vi "Check Duplicated Names.vi"(7 "Element Type":string, 8 "errors in":refnum<class "MultiErrors.lvclass">, 11 "Names":string[](array[string])) -> (0 "errors out":refnum<class "MultiErrors.lvclass">)   [LabVIEW 2020, in "VolatusConfig.lvlib"]
uses:
  VolatusConfig.lvlib
  VolatusErrorUtilities/MultiErrors/MultiErrors.lvclass
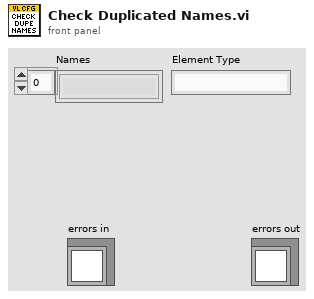
[diagram p1: front panel]
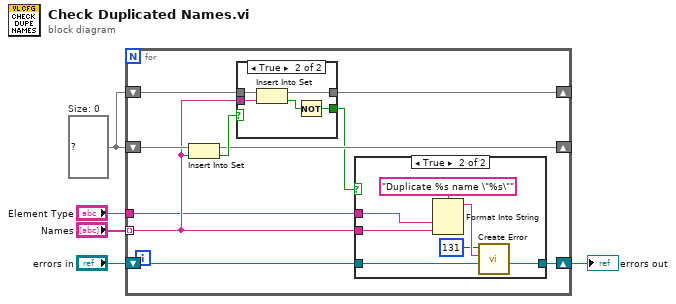
[diagram p0: block diagram]
diagram:
  w5 = set{string} {}  # Size: 0
  n1 = for {
    shift-right: [w13] -> _
    shift-left: w5 -> [w15]
    shift-right: [w11] -> _
    shift-left: w5 -> [w12]
    shift-right: [w9] -> w3
    shift-left: "errors in" -> [w10]
    tunnel: "Names" -> [w7] mode=indexing
    tunnel: "Element Type" -> [w6]
    n2 = Insert Into Set(10:w7, 11:w15) -> (2:w14:bool, 3:w13:set{string})
    n3 = case shown="True" w14 {
      tunnel: w12 -> [w16 w21]
      tunnel: w7 -> [_ w20]
      tunnel: [w16 w19] -> w11
      tunnel: [_ w17] -> w8
      frame False {
      }
      frame True {
        n4 = Insert Into Set(10:w20, 11:w21) -> (2:w18:bool, 3:w19:set{string})
        n5 = Not(x=w18) -> (.not. x?=w17:bool)
      }
    }
    n6 = case shown="True" w8 {
      tunnel: w10 -> [w22 w29]
      tunnel: [w22 w28] -> w9
      tunnel: w7 -> [_ w24]
      tunnel: w6 -> [_ w23]
      frame False {
      }
      frame True {
        n7 = Format Into String(format string="Duplicate %s name \"%s\"", w23, w24) -> (resulting string=w26:string)  [unwired: 2 in, 1 out]
        n8 = call "Create Error.vi"("MultiErrors in"=w29, "Message"=w26, "Code"=131) -> ("MultiErrors out"=w28:refnum<class "MultiErrors.lvclass">)  [unwired: 8 in]
      }
    }
  }
  "errors out" <- w3
